vi "Servo input.vi"(7 "Stop? (F)":bool, 8 "error in (no error)":errorcluster, 10 "PWM Range":cluster{"High PW":dbl, "Low PW":dbl}={"High PW"=5.8, "Low PW"=5.0}, 11 "Servo Input":dbl) -> (0 "error out":errorcluster)   [LabVIEW 2020]
uses:
  Controls/HW States.ctl
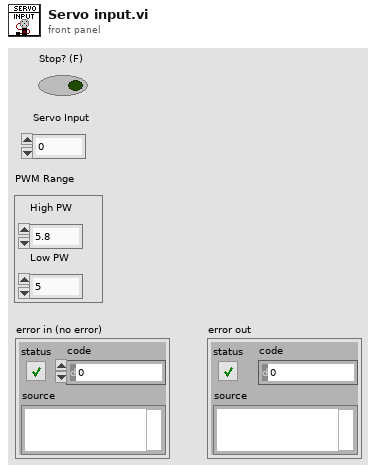
[diagram p1: front panel]
types:
  T1 = typedef "HW States.ctl" = enum16{"Initialize", "Input LED", "Input PWM", "Acquire Voltage", "Acquire Image", "Stop"}
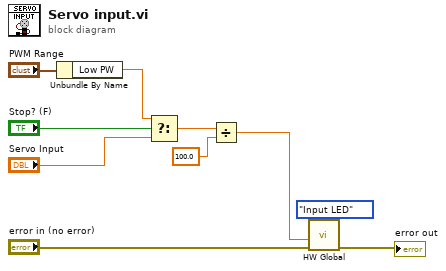
[diagram p0: block diagram]
diagram:
  n1 = Unbundle By Name("PWM Range") -> ("Low PW"=w5:dbl)
  n2 = Select(t=w5, s="Stop? (F)", f="Servo Input") -> (s? t:f=w3:dbl)
  n3 = Divide(x=w3, y=100.0) -> (x/y=w2:dbl)
  n4 = call "HW Global.vi"("HW State"=HW_States."Input LED", "error in (no error)"="error in (no error)", "servo duty cycle"=w2) -> ("error out"=→"error out":errorcluster)  [unwired: 5 in, 3 out]
